vi "getInheritanceChain.vi"(8 "error in (no error)":errorcluster, 11 "PriorityQueue in":refnum<class "PriorityQueue.lvclass">) -> (0 "error out":errorcluster, 2 "Inheritance Chain":string[](array[string]), 3 "PriorityQueue out":refnum<class "PriorityQueue.lvclass">)   [LabVIEW 2009, in "PriorityQueue.lvclass"]
doc: "Returns the inheritance chain."
uses:
  PriorityQueue.lvclass
  LinkedList/LinkedList.lvclass
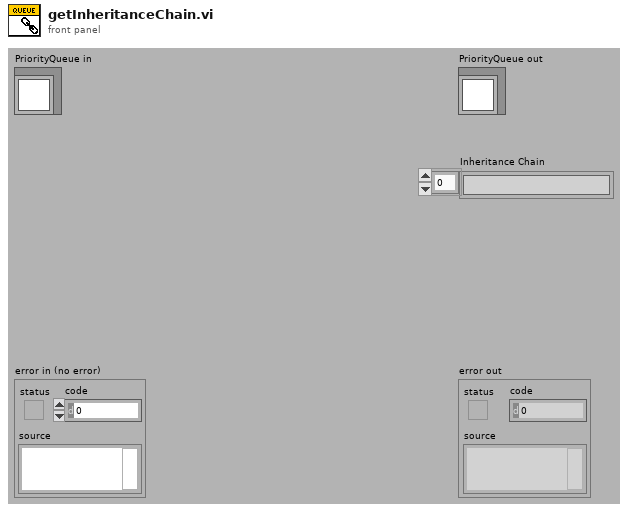
[diagram p1: front panel]
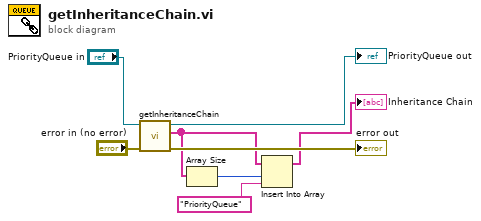
[diagram p0: block diagram]
diagram:
  n1 = call-parent "getInheritanceChain.vi"("error in (no error)"="error in (no error)", "LinkedList in"="PriorityQueue in") -> ("error out"=→"error out":errorcluster, "Inheritance Chain"=w3:string[], "LinkedList out"=→"PriorityQueue out":refnum<class "PriorityQueue.lvclass">)  [unwired: 7 in]
  n2 = Array Size(array=w3) -> (size(s)=w4:i32)
  n3 = Insert Into Array(array=w3, index=w4, new element="PriorityQueue" ("new element/subarray")) -> (→"Inheritance Chain":string[])
